vi "CelsiusToFar.vi"() -> ()   [LabVIEW 2020]
panel:
  out "Tf":dbl
  in  "Tc":dbl
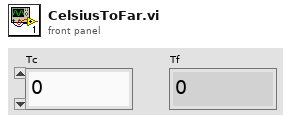
[diagram p1: front panel]
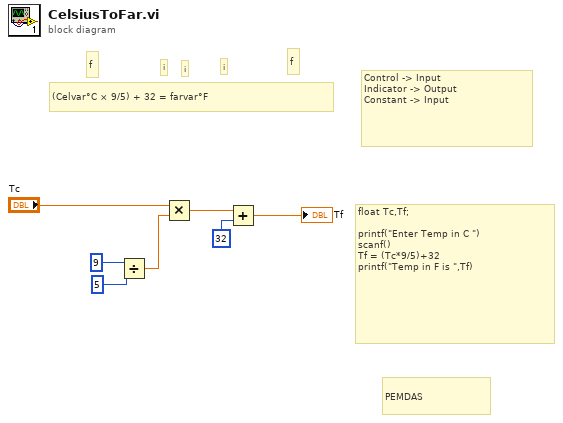
[diagram p0: block diagram]
diagram:
  # "PEMDAS"
  # "float Tc,Tf;\n\nprintf(\"Enter Temp in C \")\nscanf()\nTf = (Tc*9/5)+32\nprintf(\"Temp in F is \",Tf)"
  # "Control -> Input\nIndicator -> Output\nConstant -> Input"
  # "i"
  # "i"
  # "i"
  # "f"
  # "f"
  # "(Celvar°C × 9/5) + 32 = farvar°F"
  n1 = Divide(x=u8 9, y=u8 5) -> (x/y=w5:dbl)
  n2 = Multiply(x="Tc", y=w5) -> (x*y=w3:dbl)
  n3 = Add(x=w3, y=u8 32) -> (x+y=→"Tf":dbl)
